vi "_builtins_icon_text_add.vi"(6 "Color":u32(colorbox), 8 "Top":i32, 9 "Justify":enum8{"center", "left", "right"}(ring), 10 "Text":string, 11 "Image in":u32[][](array[numeric]) format="%08x") -> (3 "Image out":u32[][](array[numeric]) format="%08x")   [LabVIEW 2019, in "Script.lvlib"]
doc: "Adds text to the icon.\n\nCreated by: Ryan Pacini"
uses:
  Script.lvlib
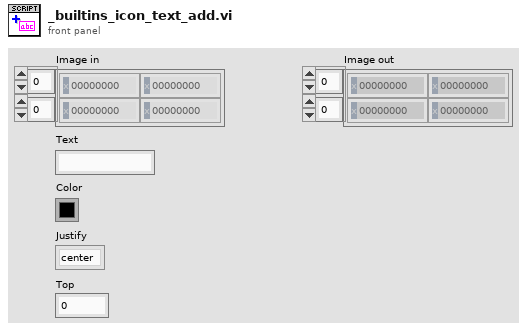
[diagram p1: front panel]
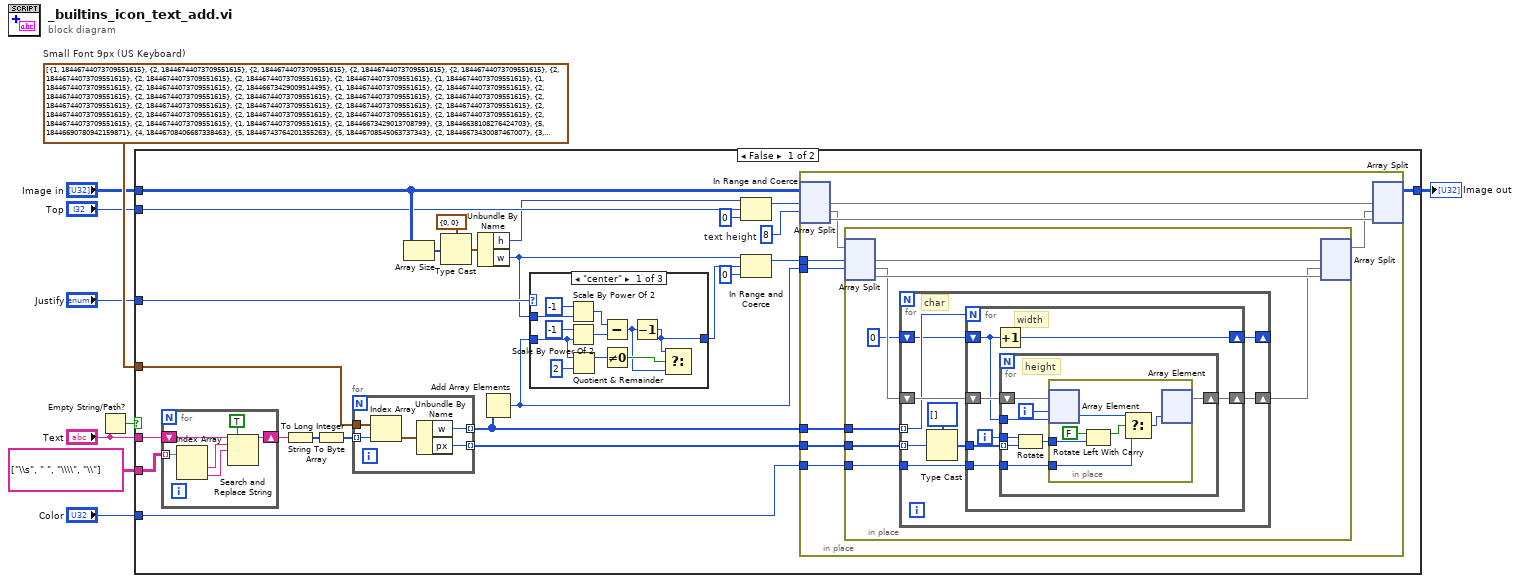
[diagram p0: block diagram]
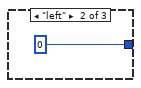
[diagram p2: hidden frame]
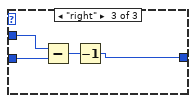
[diagram p3: hidden frame]
diagram:
  w9 = cluster{"w":i32, "px":u64}[] [{"w"=1, "px"=18446744073709551615}, {"w"=2, "px"=18446744073709551615}, {"w"=2, "px"=18446744073709551615}, {"w"=2, "px"=18446744073709551615}, {"w"=2, "px"=18446744073709551615}, {"w"=2, "px"=18446744073709551615}, {"w"=2, "px"=18446744073709551615}, {"w"=2, "px"=18446744073709551615}, {"w"=2, "px"=18446744073709551615}, {"w"=1, "px"=18446744073709551615}, {"w"=1, "px"=18446744073709551615}, {"w"=2, "px"=18446744073709551615}, {"w"=2, "px"=18446673429009514495}, {"w"=1, "px"=18446744073709551615}, {"w"=2, "px"=18446744073709551615}, {"w"=2, "px"=18446744073709551615}, {"w"=2, "px"=18446744073709551615}, {"w"=2, "px"=18446744073709551615}, {"w"=2, "px"=18446744073709551615}, {"w"=2, "px"=18446744073709551615}, {"w"=2, "px"=18446744073709551615}, {"w"=2, "px"=18446744073709551615}, {"w"=2, "px"=18446744073709551615}, {"w"=2, "px"=18446744073709551615}, {"w"=2, "px"=18446744073709551615}, {"w"=2, "px"=18446744073709551615}, {"w"=2, "px"=18446744073709551615}, {"w"=2, "px"=18446744073709551615}, {"w"=2, "px"=18446744073709551615}, {"w"=2, "px"=18446744073709551615}, {"w"=2, "px"=18446744073709551615}, {"w"=2, "px"=18446744073709551615}, {"w"=1, "px"=18446744073709551615}, {"w"=2, "px"=18446673429013708799}, {"w"=3, "px"=18446638108276424703}, {"w"=5, "px"=18446690780942159871}, {"w"=4, "px"=18446708406687338463}, {"w"=5, "px"=18446743764201355263}, {"w"=5, "px"=18446708545063737343}, {"w"=2, "px"=18446673430087467007}, {"w"=3, "px"=18446708613381603295}, {"w"=3, "px"=18446673566987444159}, {"w"=3, "px"=18446638108276424703}, {"w"=4, "px"=18446743934389452799}, {"w"=2, "px"=18446744073709535167}, {"w"=3, "px"=18446744072098938879}, {"w"=2, "px"=18446744073709535231}, {"w"=3, "px"=18446708750283685887}, {"w"=4, "px"=18446708544392650751}, {"w"=3, "px"=18446708476481626111}, {"w"=4, "px"=18446638451332714495}, {"w"=4, "px"=18446638451335864319}, {"w"=4, "px"=18446726274015555583}, {"w"=4, "px"=18446620651649212415}, {"w"=4, "px"=18446708612843692031}, {"w"=4, "px"=18446620859148787711}, {"w"=4, "px"=18446708545197957119}, {"w"=4, "px"=18446708543859974143}, {"w"=2, "px"=18446744072635793407}, {"w"=2, "px"=18446744072635793343}, {"w"=3, "px"=18446744073168478207}, {"w"=3, "px"=18446744073703260159}, {"w"=3, "px"=18446744072633696255}, {"w"=3, "px"=18446673566452662271}, {"w"=7, "px"=18446717529295544295}, {"w"=5, "px"=18446691089777145855}, {"w"=5, "px"=18446620617285799935}, {"w"=5, "px"=18446690986835300351}, {"w"=5, "px"=18446620617956888575}, {"w"=4, "px"=18446620651914498047}, {"w"=4, "px"=18446620651914510335}, {"w"=5, "px"=18446682224699361279}, {"w"=5, "px"=18446664597616703487}, {"w"=2, "px"=18446673429009514495}, {"w"=4, "px"=18446726412530327551}, {"w"=5, "px"=18446664563659094015}, {"w"=4, "px"=18446673429009502207}, {"w"=6, "px"=18446668841648634879}, {"w"=5, "px"=18446664460714620927}, {"w"=5, "px"=18446690986701082623}, {"w"=5, "px"=18446620617286336511}, {"w"=5, "px"=18446690986700560383}, {"w"=5, "px"=18446620617285810175}, {"w"=5, "px"=18446682225374629887}, {"w"=4, "px"=18446620790429310975}, {"w"=5, "px"=18446664598422015999}, {"w"=4, "px"=18446655767837663231}, {"w"=6, "px"=18446668944729692159}, {"w"=4, "px"=18446655768639811583}, {"w"=4, "px"=18446655768642969599}, {"w"=4, "px"=18446620859146670079}, {"w"=3, "px"=18446638244637425567}, {"w"=3, "px"=18446673428474748927}, {"w"=3, "px"=18446638382615355295}, {"w"=4, "px"=18446708545740079103}, {"w"=4, "px"=18446744073709551375}, {"w"=3, "px"=18446673567526420479}, {"w"=4, "px"=18446744072898990079}, {"w"=4, "px"=18446673428471586815}, {"w"=4, "px"=18446744072900038655}, {"w"=4, "px"=18446726411993468927}, {"w"=4, "px"=18446744073167413247}, {"w"=3, "px"=18446708612844732415}, {"w"=4, "px"=18446744072898990063}, {"w"=4, "px"=18446673428471590911}, {"w"=2, "px"=18446673703887421439}, {"w"=2, "px"=18446673703887421375}, {"w"=4, "px"=18446673428738977791}, {"w"=2, "px"=18446673429009514495}, {"w"=6, "px"=18446744071690759167}, {"w"=4, "px"=18446744072093675519}, {"w"=4, "px"=18446744071825231871}, {"w"=4, "px"=18446744072093671359}, {"w"=4, "px"=18446744072898990063}, {"w"=3, "px"=18446744072094728191}, {"w"=3, "px"=18446744072094695423}, {"w"=3, "px"=18446743797216829439}, {"w"=4, "px"=18446744072362119167}, {"w"=4, "px"=18446744072362123263}, {"w"=5, "px"=18446744072496842751}, {"w"=4, "px"=18446744072365256703}, {"w"=4, "px"=18446744072365268927}, {"w"=4, "px"=18446744071828377599}, {"w"=3, "px"=18446708750820564959}, {"w"=2, "px"=18446673429009514495}, {"w"=3, "px"=18446673429548482495}, {"w"=4, "px"=18446690884834557951}, {"w"=2, "px"=18446673429009514495}, {"w"=2, "px"=18446673429009514495}, {"w"=0, "px"=18446744073709551615}, {"w"=2, "px"=18446744073709535167}, {"w"=4, "px"=18446691157831311295}, {"w"=3, "px"=18446744073709510495}, {"w"=5, "px"=18446744073709508607}, {"w"=4, "px"=18446708407762149343}, {"w"=4, "px"=18446708407762128863}, {"w"=4, "px"=18446708545740079103}, {"w"=6, "px"=18446699748771998719}, {"w"=5, "px"=15559874864230141951}, {"w"=3, "px"=18446744073168478207}, {"w"=6, "px"=18446607389188654079}, {"w"=0, "px"=18446744073709551615}, {"w"=2, "px"=18446673429009514495}, {"w"=0, "px"=18446744073709551615}, {"w"=0, "px"=18446744073709551615}, {"w"=2, "px"=18446673704965373951}, {"w"=2, "px"=18446673704965373951}, {"w"=3, "px"=18446638520593285119}, {"w"=3, "px"=18446638520593285119}, {"w"=3, "px"=18446744072092647423}, {"w"=4, "px"=18446744073702211583}, {"w"=6, "px"=18446744073701425151}, {"w"=4, "px"=18446690884834557951}, {"w"=6, "px"=18446475396326096895}, {"w"=3, "px"=18446568150234251263}, {"w"=3, "px"=18446744072633696255}, {"w"=6, "px"=18446744072764508159}, {"w"=0, "px"=18446744073709551615}, {"w"=2, "px"=18446673429009514495}, {"w"=4, "px"=12682048245608734719}, {"w"=1, "px"=18446744073709551615}, {"w"=2, "px"=18446743798827433919}, {"w"=4, "px"=18446744004180561887}, {"w"=4, "px"=18446726342203396095}, {"w"=4, "px"=18446655973998198783}, {"w"=4, "px"=18446655631198773247}, {"w"=2, "px"=18446673429009514431}, {"w"=4, "px"=18446690883489222559}, {"w"=3, "px"=18446638520593285119}, {"w"=5, "px"=18446690917446320127}, {"w"=2, "px"=18446673430087467007}, {"w"=3, "px"=18446744073168478207}, {"w"=4, "px"=18446744073702207487}, {"w"=2, "px"=18446744073705357311}, {"w"=5, "px"=18446690848995278847}, {"w"=4, "px"=18446480190918885375}, {"w"=2, "px"=18446743798831644671}, {"w"=3, "px"=18446744072092622847}, {"w"=2, "px"=18446673430087467007}, {"w"=2, "px"=18446743797757902847}, {"w"=2, "px"=18446673155209560063}, {"w"=4, "px"=18446744071014657919}, {"w"=3, "px"=18446743659779973087}, {"w"=2, "px"=18446744072635809791}, {"w"=2, "px"=18446744073709535039}, {"w"=2, "px"=18446743797757902847}, {"w"=2, "px"=18446743797757902847}, {"w"=3, "px"=18446744072633696255}, {"w"=5, "px"=18446743763127089151}, {"w"=5, "px"=18446743763127089151}, {"w"=5, "px"=18446743763127089151}, {"w"=3, "px"=18446743936268484575}, {"w"=4, "px"=18428694145881059327}, {"w"=4, "px"=18442204944763170815}, {"w"=4, "px"=18437701345135800319}, {"w"=4, "px"=18437701345135800319}, {"w"=4, "px"=18424190546253688831}, {"w"=4, "px"=18437701345135800319}, {"w"=6, "px"=18446713079674676223}, {"w"=5, "px"=18446690986835300335}, {"w"=4, "px"=18428606253136580607}, {"w"=4, "px"=18442117052018692095}, {"w"=4, "px"=18437613452391321599}, {"w"=4, "px"=18424102653509210111}, {"w"=2, "px"=18410644906868457471}, {"w"=3, "px"=18437666504632680447}, {"w"=3, "px"=18428553752261672959}, {"w"=3, "px"=18401707801479987199}, {"w"=4, "px"=18446638173500973055}, {"w"=5, "px"=18433153661832509439}, {"w"=5, "px"=18437683787446341631}, {"w"=5, "px"=18442187387073712127}, {"w"=5, "px"=18433180187818971135}, {"w"=5, "px"=18433180187818971135}, {"w"=5, "px"=18426424788377915391}, {"w"=4, "px"=18446743729570054143}, {"w"=5, "px"=18446682121349599231}, {"w"=5, "px"=18437657399167275007}, {"w"=5, "px"=18442160998794645503}, {"w"=5, "px"=18433153799539904511}, {"w"=5, "px"=18433153799539904511}, {"w"=4, "px"=18437648569388228607}, {"w"=4, "px"=18446673222579503103}, {"w"=4, "px"=18446708543855763455}, {"w"=4, "px"=18446708819807424511}, {"w"=4, "px"=18446726343273992191}, {"w"=4, "px"=18446691296340856831}, {"w"=4, "px"=18446691296340856831}, {"w"=4, "px"=18446656111968767999}, {"w"=4, "px"=18446708888526901247}, {"w"=6, "px"=18446744072764507135}, {"w"=4, "px"=18446744072900038639}, {"w"=4, "px"=18446673565910552575}, {"w"=4, "px"=18446708612843687935}, {"w"=4, "px"=18446708544124211199}, {"w"=4, "px"=18446656111163461631}, {"w"=2, "px"=18446603061339078655}, {"w"=3, "px"=18446708614455345151}, {"w"=3, "px"=18446673017766395903}, {"w"=3, "px"=18446743386510573567}, {"w"=3, "px"=18446743798288457727}, {"w"=4, "px"=18446638518977409023}, {"w"=4, "px"=18446673565642100735}, {"w"=4, "px"=18446726342200233983}, {"w"=4, "px"=18446708543855759359}, {"w"=4, "px"=18446691295267098623}, {"w"=4, "px"=18446656110895009791}, {"w"=4, "px"=18446744073165332479}, {"w"=4, "px"=18446744071823134719}, {"w"=4, "px"=18446673566178988031}, {"w"=4, "px"=18446726342737121279}, {"w"=4, "px"=18446708544392646655}, {"w"=4, "px"=18446656111431897087}, {"w"=4, "px"=18446726342740271039}, {"w"=4, "px"=18446673428471586751}, {"w"=4, "px"=18446656111435046847}]  # Small Font 9px (US Keyboard)
  n1 = Empty String/Path?(string/path="Text") -> (empty?=w3:bool)
  n2 = case shown="False" w3 {
    tunnel: "Text" -> [w12 _]
    tunnel: w9 -> [w32 _]
    tunnel: "Image in" -> [w28 w109]
    tunnel: [w27 w109] -> w7
    tunnel: "Top" -> [w21 _]
    tunnel: "Justify" -> [w19 _]
    tunnel: "Color" -> [w14 _]
    tunnel: string[][] [["\\s", " "], ["\\\\", "\\"]] ("escape chars (\\\\, \\s)") -> [w11 _]
    frame False {
      w26 = 8  # text height
      n3 = for {
        shift-right: [w40] -> w13
        shift-left: w12 -> [w38]
        tunnel: w11 -> [w37] mode=indexing
        n4 = Index Array(array=w37) -> (element #1=w36:string, element #2=w35:string)  [unwired: 2 in]
        n5 = Search and Replace String(replace all?=TRUE ("replace all? (F)"), input string=w38, search string=w36, replace string=w35) -> (result string=w40:string)  [unwired: 4 in, 3 out]
      }
      n6 = String To Byte Array(string=w13) -> (unsigned byte array=w34:u8[])
      n7 = To Long Integer(number=w34) -> (32bit integer=w33:i32[])
      n8 = for {
        tunnel: w33 -> [w108] mode=indexing
        tunnel: w32 -> [w107]
        tunnel: [w105] -> w16 mode=indexing
        tunnel: [w104] -> w15 mode=indexing
        n9 = Index Array(array=w107, index=w108) -> (element=w106:cluster{"w":i32, "px":u64})
        n10 = Unbundle By Name(w106) -> ("w"=w105:i32, "px"=w104:u64)
      }
      n11 = Array Size(array=w28) -> (size(s)=w31:i32[])
      n12 = Type Cast(type=cluster{"h":i32, "w":i32} {"h"=0, "w"=0} ("size"), x=w31) -> (*(type *) &x=w29:cluster{"h":i32, "w":i32})
      n13 = Unbundle By Name(w29) -> ("h"=w20:i32, "w"=w18:i32)
      n14 = Add Array Elements(numeric array=w16) -> (sum=w10:i32)
      n15 = case shown="\"center\"" w19 {
        tunnel: w18 -> [w49 _ w56]
        tunnel: [w41 0 ("lower limit") w53] -> w17
        tunnel: w10 -> [w44 _ w54]
        frame "center" {
          n16 = Scale By Power Of 2(n=i16 -1, x=w49) -> (x*2^n=w48:i32)
          n17 = Scale By Power Of 2(n=i16 -1, x=w44) -> (x*2^n=w47:i32)
          n18 = Quotient & Remainder(x=w44, y=2) -> (x-y*floor(x/y)=w46:i32)  [unwired: 1 out]
          n19 = Subtract(x=w48, y=w47) -> (x-y=w42:i32)
          n20 = Not Equal To 0?(x=w46) -> (x != 0?=w43:bool)
          n21 = Decrement(x=w42) -> (x-1=w41:i32)
          n22 = Select(t=w41, s=w43, f=w42) -> ()  [unwired: 1 out]
        }
        frame "left" {
        }
        frame "right" {
          n23 = Subtract(x=w56, y=w54) -> (x-y=w55:i32)
          n24 = Decrement(x=w55) -> (x-1=w53:i32)
        }
      }
      n25 = In Range and Coerce(upper limit=w20, x=w21, lower limit=0) -> (coerced(x)=w22:i32)  [unwired: 1 out]
      n26 = In Range and Coerce(upper limit=w18, x=w17, lower limit=0) -> (coerced(x)=w24:i32)  [unwired: 1 out]
      n27 = in-place {
        in-place-border: w24 -> [w62]
        in-place-border: w10 -> [w60]
        in-place-border: w16 -> [w59]
        in-place-border: w15 -> [w58]
        in-place-border: w14 -> [w57]
        n28 = in-place-split #1(w28, w22, w26) -> (w64:u32[][], w63:u32[][], w65:u32[][])
        n29 = in-place {
          in-place-border: w59 -> [w68]
          in-place-border: w58 -> [w70]
          in-place-border: w57 -> [w67]
          n30 = in-place-split #2(w63, w62, w60) -> (w73:u32[][], w71:u32[][], w72:u32[][])
          n31 = for {
            tunnel: w70 -> [w80] mode=indexing
            shift-right: [w81] -> w69
            shift-left: w71 -> [w82]
            tunnel: w68 -> [w77] mode=indexing
            tunnel: w67 -> [w76]
            shift-right: [w74] -> _
            shift-left: 0 -> [w75]
            # "char"
            n32 = Type Cast(type=u8[] [], x=w80) -> (*(type *) &x=w78:u8[])
            n33 = for {
              N: w77 -> [_]
              shift-right: [w88] -> w81
              shift-left: w82 -> [w89]
              tunnel: w78 -> [w87]
              shift-right: [w84] -> w74
              shift-left: w75 -> [w85]
              tunnel: w76 -> [w86]
              i -> [w83]
              # "width"
              n34 = Increment(x=w85) -> (x+1=w84:i32)
              n35 = for {
                shift-right: [w94] -> w88
                shift-left: w89 -> [w97]
                tunnel: w87 -> [w92] mode=indexing
                tunnel: w85 -> [w93]
                tunnel: w86 -> [w95]
                tunnel: w83 -> [w90]
                i -> [w96]
                # "height"
                n36 = Rotate(1:w92, 2:w90) -> (0:w91:u8)
                n37 = in-place {
                  in-place-border: w95 -> [w101]
                  in-place-border: w91 -> [w98]
                  n38 = in-place-array #3(w97, w96, w93) -> (w100:u32)
                  n39 = Rotate Left With Carry(2:w98, 3:FALSE ("carry")) -> (1:w102:bool)  [unwired: 1 out]
                  n40 = Select(t=w100, s=w102, f=w101) -> (s? t:f=w99:u32)
                  n41 = in-place-array #3(w99) -> (w94:u32[][])  [unwired: 2 out]
                }
              }
            }
          }
          n42 = in-place-split #2(w73, w69, w72) -> (w61:u32[][])  [unwired: 2 out]
        }
        n43 = in-place-split #1(w64, w61, w65) -> (w27:u32[][])  [unwired: 2 out]
      }
    }
    frame True {
    }
  }
  "Image out" <- w7
